vi "ParseAllVarsFile.vi"(8 "Path":path) -> (0 "CA input vars":T1, 1 "SCM input vars":T1, 2 "VP input vars":T1, 3 "CA output vars":T2, 4 "VP output vars":T2, 5 "VM output vars":T2, 6 "SCM output vars":T2, 7 "VM input vars":T1)   [LabVIEW 2019]
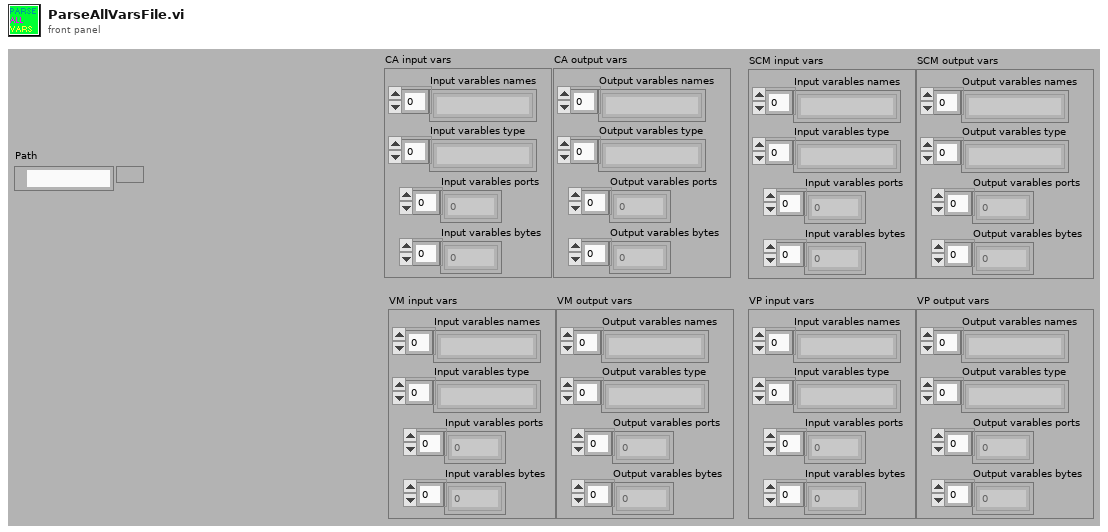
[diagram p1: front panel]
types:
  T1 = cluster{"Input varables names":string[], "Input varables type":string[], "Input varables ports":i32[], "Input varables bytes":i32[]}
  T2 = cluster{"Output varables names":string[], "Output varables type":string[], "Output varables ports":i32[], "Output varables bytes":i32[]}
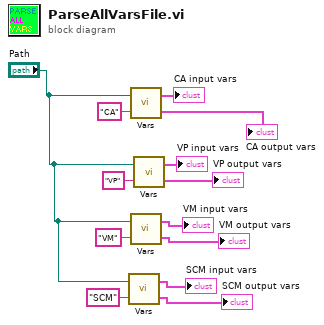
[diagram p0: block diagram]
diagram:
  n1 = call "Vars.vi"("name or relative path"="SCM", "Path"="Path") -> ("output"=→"SCM output vars":T2, "input"=→"SCM input vars":T1)
  n2 = call "Vars.vi"("name or relative path"="CA", "Path"="Path") -> ("output"=→"CA output vars":T2, "input"=→"CA input vars":T1)
  n3 = call "Vars.vi"("name or relative path"="VM", "Path"="Path") -> ("output"=→"VM output vars":T2, "input"=→"VM input vars":T1)
  n4 = call "Vars.vi"("name or relative path"="VP", "Path"="Path") -> ("output"=→"VP output vars":T2, "input"=→"VP input vars":T1)
